vi "FIFOStart.vi"(1 "Set/Get":bool, 2 "Start (input)":dbl format="%.2f") -> (0 "Start (output)":dbl format="%.2f")   [LabVIEW 2009]
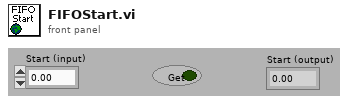
[diagram p1: front panel]
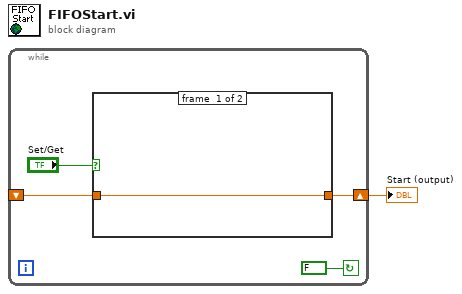
[diagram p0: block diagram]
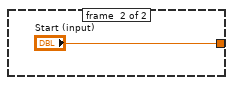
[diagram p2: hidden frame]
diagram:
  n1 = while {
    shift-right: [w4] -> w1
    shift-left: _ -> [w3]
    stop <- FALSE continue-if-true
    n2 = case shown="True" "Set/Get" {
      tunnel: [w6 "Start (input)"] -> w4
      tunnel: w3 -> [w6 _]
      frame #0 {
      }
      frame #1 {
      }
    }
  }
  "Start (output)" <- w1
